vi "LuaVIEW Pushing and Pulling.vi"() -> (0 "pass?":bool)   [LabVIEW 2012]
uses:
  typedefs/t_LuaVIEW Reference.ctl
  subvis/private/LuaVIEW Pull (boolean).vi
  subvis/private/LuaVIEW Push (boolean).vi
  subvis/private/LuaVIEW Pull (number).vi
  subvis/private/LuaVIEW Push (number).vi
  subvis/private/LuaVIEW Pull (string).vi
  subvis/private/LuaVIEW Push (string).vi
  subvis/private/LuaVIEW Pull (path).vi
  subvis/private/LuaVIEW Push (path).vi
  subvis/private/LuaVIEW Pull (U32).vi
  subvis/private/LuaVIEW Push (object).vi
  subvis/private/LuaVIEW Pull (object).vi
  subvis/private/LuaVIEW Push (U32).vi
  subvis/private/LuaVIEW Push (refnum).vi
  subvis/private/LuaVIEW Pull (refnum).vi
  subvis/private/LuaVIEW Pull (I8).vi
  subvis/private/LuaVIEW Push (I8).vi
  subvis/private/LuaVIEW Pull (U8).vi
  subvis/private/LuaVIEW Push (U8).vi
  subvis/private/LuaVIEW Pull (I16).vi
  subvis/private/LuaVIEW Push (I16).vi
  subvis/private/LuaVIEW Pull (U16).vi
  subvis/private/LuaVIEW Push (U16).vi
  subvis/private/LuaVIEW Pull (I32).vi
  subvis/private/LuaVIEW Push (I32).vi
panel:
  in  "script file":path=path "scripts/push pull test.lua"
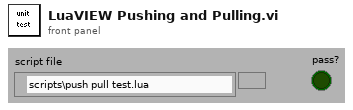
[diagram p1: front panel]
types:
  T1 = enum32{"execute", "initialize", "bool:b=pass_boolean(bool:b)", "pull_boolean(any:value)", "num:n=pass_number(num:n)", "pull_number(any:value)", "str:s=pass_string(str:s)", "pull_string(any:value)", "str:s=pass_path(str:s)", "pull_path(any:value)", "obj:o=push_object(U32:u,str:methodtable)", "U32:u=pull_object(any:value)", "bool:already_dead=kill_object(obj:o)", "any:attribute=get_object_attribute(str:key,obj:o)", "set_object_attribute(str:key,obj:o,any:value)", "any:attribute=unchecked_goa(any:key,...)", "unchecked_soa(any:key,...)", "ref:r=push_refnum(U32:u)", "U32:u=pull_refnum(any:value)", "I8:n=pass_I8(I8:n)", "pull_I8(any:value)", "U8:n=pass_U8(U8:n)", "pull_U8(any:value)", "I16:n=pass_I16(I16:n)", "pull_I16(any:value)", "U16:n=pass_U16(U16:n)", "pull_U16(any:value)", "I32:n=pass_I32(I32:n)", "pull_I32(any:value)", "U32:n=pass_U32(U32:n)", "pull_U32(any:value)", "str:buf=dump()", "str:new,I32:index=poll(I32:index)", "cleanup"}
  T2 = typedef "t_LuaVIEW Reference.ctl" = refnum<k1>
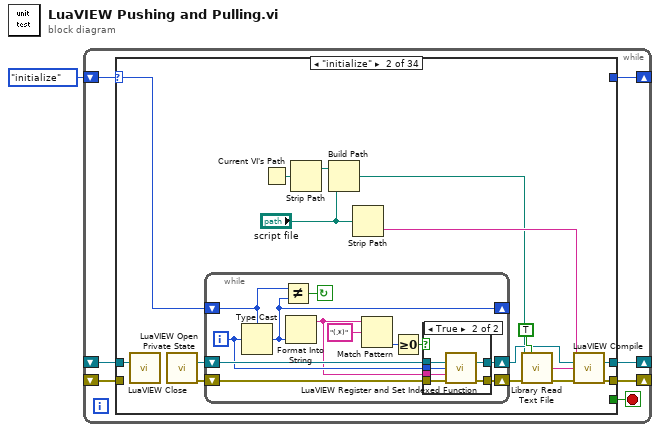
[diagram p0: block diagram]
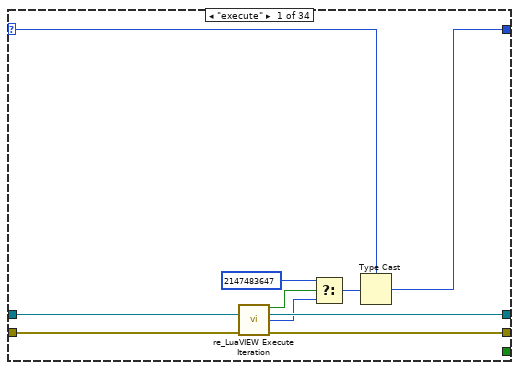
[diagram p2: hidden frame]
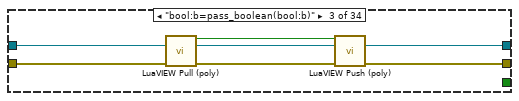
[diagram p4: hidden frame]
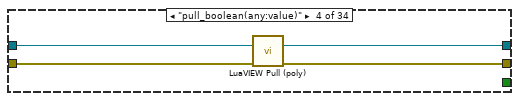
[diagram p5: hidden frame]
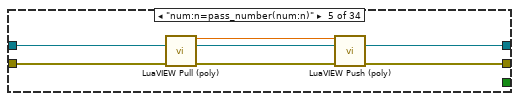
[diagram p6: hidden frame]
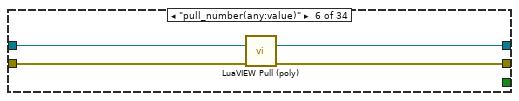
[diagram p7: hidden frame]
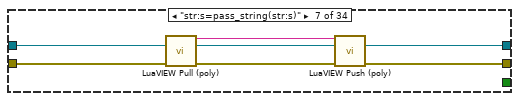
[diagram p8: hidden frame]
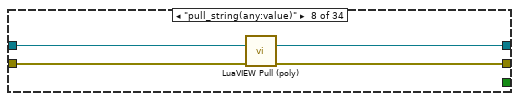
[diagram p9: hidden frame]
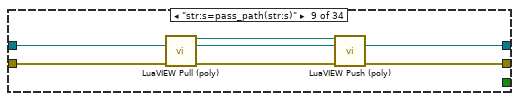
[diagram p10: hidden frame]
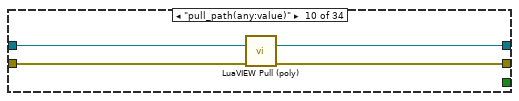
[diagram p11: hidden frame]
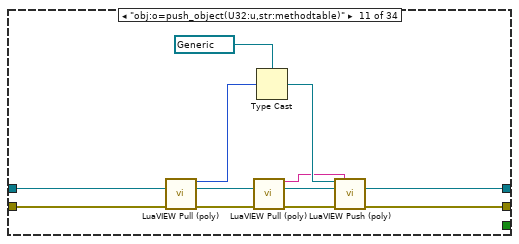
[diagram p12: hidden frame]
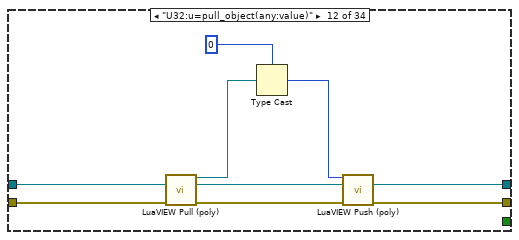
[diagram p13: hidden frame]
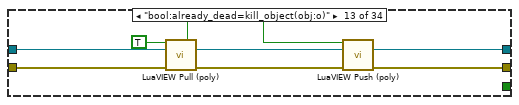
[diagram p14: hidden frame]
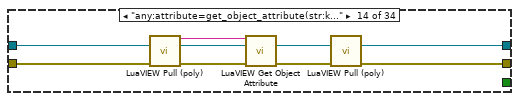
[diagram p15: hidden frame]
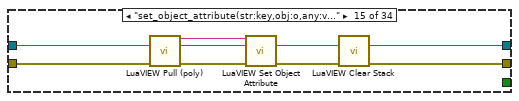
[diagram p16: hidden frame]
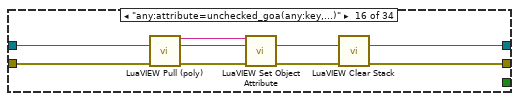
[diagram p17: hidden frame]
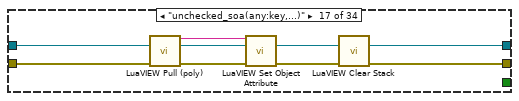
[diagram p18: hidden frame]
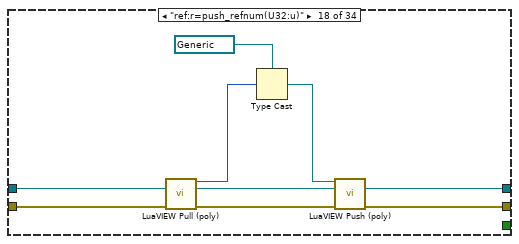
[diagram p19: hidden frame]
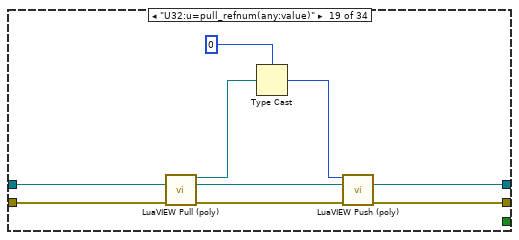
[diagram p20: hidden frame]
diagram:
  n1 = while {
    shift-right: [w6] -> _
    shift-left: T1."initialize" -> [w8]
    shift-right: [w4] -> _
    shift-left: _ -> [w5]
    shift-right: [w3] -> _
    shift-left: _ -> [w2]
    stop <- w7 stop-if-true
    n2 = case shown="\"initialize\"" w8 {
      selector: w8 -> [w11 w30 _ _ _ _ _ _ _ _ _ _ _ _ _ _ _ _ _ _ _ _ _ _ _ _ _ _ _ _ _ _ _ _]
      tunnel: [_ _ _ _ _ _ _ _ _ _ _ _ _ _ _ _ _ _ _ _ _ _ _ _ _ _ _ _ _ _ _ _ _ TRUE] -> w7
      tunnel: [w9 _ _ _ _ _ _ _ _ _ _ _ _ _ _ _ _ _ _ _ _ _ _ _ _ _ _ _ _ _ _ _ _ _] -> w6
      tunnel: w5 -> [w18 w34 w60 w64 w71 w75 w82 w86 w93 w97 w107 w118 w126 w135 w144 w153 w162 w169 w180 w187 w191 w198 w202 w209 w213 w220 w224 w231 w235 w242 w246 w254 w258 w276]
      tunnel: [w15 w31 w58 w62 w69 w73 w80 w85 w91 w96 w105 w115 w124 w128 w137 w146 w155 w166 w177 w185 w190 w196 w201 w207 w212 w218 w223 w229 w234 w240 w245 w248 w262 w275] -> w4
      tunnel: [w16 w29 w57 w63 w68 w74 w79 w84 w90 w95 w104 w114 w123 w129 w138 w147 w156 w165 w176 w184 w189 w195 w200 w206 w211 w217 w222 w228 w233 w239 w244 w251 w261 _] -> w3
      tunnel: w2 -> [w17 _ w61 w65 w72 w76 w83 w87 w94 w98 w108 w119 w127 w136 w145 w154 w163 w170 w181 w188 w192 w199 w203 w210 w214 w221 w225 w232 w236 w243 w247 w255 w260 w273]
      frame "execute" {
        n3 = call "re_LuaVIEW Execute Iteration.vi"("LuaVIEW reference in"=w18, "init or indexed function error"=w17) -> ("last?"=w13:bool, "LuaVIEW reference out"=w15:T2, "function index"=w14:i32, "final error"=w16:errorcluster)  [unwired: 10 in]
        n4 = Select(t=2147483647, s=w13, f=w14) -> (s? t:f=w10:i32)
        n5 = Type Cast(type=w11, x=w10) -> (*(type *) &x=w9:T1)
      }
      frame "initialize" {
        n6 = call "LuaVIEW Close.vi"("LuaVIEW reference"=w34) -> ()  [unwired: 14 in, 1 out]
        n7 = call "LuaVIEW Open Private State.vi"() -> ("LuaVIEW reference"=w32:T2, "error out"=w33:errorcluster)  [unwired: 14 in]
        n8 = while {
          shift-right: [w40] -> w25
          shift-left: w33 -> [w43]
          shift-right: [w41] -> w26
          shift-left: w32 -> [w42]
          shift-right: [w35] -> _
          shift-left: w30 -> [w36]
          i -> [w39]
          stop <- w46 continue-if-true
          n9 = Type Cast(type=w36, x=w39) -> (*(type *) &x=w35:T1)
          n10 = Not Equal?(x=w36, y=w35) -> (x != y?=w46:bool)
          n11 = Format Into String(w35) -> (resulting string=w37:string)  [unwired: 3 in, 1 out]
          n12 = Match Pattern(string=w37, regular expression="(.*)") -> (offset past match=w44:i32)  [unwired: 1 in, 3 out]
          n13 = Greater Or Equal To 0?(x=w44) -> (x >= 0?=w38:bool)
          n14 = case shown="True" w38 {
            tunnel: w42 -> [w48 w51]
            tunnel: w39 -> [_ w52]
            tunnel: w37 -> [_ w49]
            tunnel: [w47 w54] -> w40
            tunnel: [w48 w53] -> w41
            tunnel: w43 -> [w47 w50]
            frame False {
            }
            frame True {
              n15 = call "LuaVIEW Register and Set Indexed Function.vi"("LuaVIEW reference in"=w51, "index"=w52, "synopsis"=w49, "error in (no error)"=w50) -> ("LuaVIEW reference out"=w53:T2, "error out"=w54:errorcluster)  [unwired: 10 in]
            }
          }
        }
        n16 = Current VI's Path() -> (path=w23:path)
        n17 = Strip Path(path=w23) -> (stripped path=w22:path)  [unwired: 1 out]
        n18 = Build Path(base path=w22, name or relative path="script file") -> (appended path=w19:path)
        n19 = Strip Path(path="script file") -> (name=w20:string)  [unwired: 1 out]
        n20 = call "Library Read Text File.vi"("file path"=w19, "convert eol (F)"=TRUE, "error in (no error)"=w25) -> ("read text"=w24:string, "error out"=w27:errorcluster)  [unwired: 10 in, 1 out]
        n21 = call "LuaVIEW Compile.vi"("script name"=w20, "LuaVIEW reference in"=w26, "script"=w24, "error in (no error)"=w27) -> ("LuaVIEW reference out"=w31:T2, "error out"=w29:errorcluster)  [unwired: 10 in]
      }
      frame "bool:b=pass_boolean(bool:b)" {
        n22 = call-poly "LuaVIEW Pull (poly).vi"("LuaVIEW reference in"=w60, "error in (no error)"=w61) -> ("boolean"=w55:bool, "LuaVIEW reference out"=w56:T2, "error out"=w59:errorcluster)  [unwired: 11 in]
        n23 = call-poly "LuaVIEW Push (poly).vi"("boolean"=w55, "LuaVIEW reference in"=w56, "error in (no error)"=w59) -> ("LuaVIEW reference out"=w58:T2, "error out"=w57:errorcluster)  [unwired: 11 in]
      }
      frame "pull_boolean(any:value)" {
        n24 = call-poly "LuaVIEW Pull (poly).vi"("LuaVIEW reference in"=w64, "error in (no error)"=w65) -> ("LuaVIEW reference out"=w62:T2, "error out"=w63:errorcluster)  [unwired: 11 in, 1 out]
      }
      frame "num:n=pass_number(num:n)" {
        n25 = call-poly "LuaVIEW Pull (poly).vi"("LuaVIEW reference in"=w71, "error in (no error)"=w72) -> ("number"=w66:dbl, "LuaVIEW reference out"=w67:T2, "error out"=w70:errorcluster)  [unwired: 11 in]
        n26 = call-poly "LuaVIEW Push (poly).vi"("number"=w66, "LuaVIEW reference in"=w67, "error in (no error)"=w70) -> ("LuaVIEW reference out"=w69:T2, "error out"=w68:errorcluster)  [unwired: 11 in]
      }
      frame "pull_number(any:value)" {
        n27 = call-poly "LuaVIEW Pull (poly).vi"("LuaVIEW reference in"=w75, "error in (no error)"=w76) -> ("LuaVIEW reference out"=w73:T2, "error out"=w74:errorcluster)  [unwired: 11 in, 1 out]
      }
      frame "str:s=pass_string(str:s)" {
        n28 = call-poly "LuaVIEW Pull (poly).vi"("LuaVIEW reference in"=w82, "error in (no error)"=w83) -> ("string"=w77:string, "LuaVIEW reference out"=w78:T2, "error out"=w81:errorcluster)  [unwired: 11 in]
        n29 = call-poly "LuaVIEW Push (poly).vi"("string"=w77, "LuaVIEW reference in"=w78, "error in (no error)"=w81) -> ("LuaVIEW reference out"=w80:T2, "error out"=w79:errorcluster)  [unwired: 11 in]
      }
      frame "pull_string(any:value)" {
        n30 = call-poly "LuaVIEW Pull (poly).vi"("LuaVIEW reference in"=w86, "error in (no error)"=w87) -> ("LuaVIEW reference out"=w85:T2, "error out"=w84:errorcluster)  [unwired: 11 in, 1 out]
      }
      frame "str:s=pass_path(str:s)" {
        n31 = call-poly "LuaVIEW Pull (poly).vi"("LuaVIEW reference in"=w93, "error in (no error)"=w94) -> ("path"=w88:path, "LuaVIEW reference out"=w89:T2, "error out"=w92:errorcluster)  [unwired: 11 in]
        n32 = call-poly "LuaVIEW Push (poly).vi"("path"=w88, "LuaVIEW reference in"=w89, "error in (no error)"=w92) -> ("LuaVIEW reference out"=w91:T2, "error out"=w90:errorcluster)  [unwired: 11 in]
      }
      frame "pull_path(any:value)" {
        n33 = call-poly "LuaVIEW Pull (poly).vi"("LuaVIEW reference in"=w97, "error in (no error)"=w98) -> ("LuaVIEW reference out"=w96:T2, "error out"=w95:errorcluster)  [unwired: 11 in, 1 out]
      }
      frame "obj:o=push_object(U32:u,str:methodtable)" {
        n34 = call-poly "LuaVIEW Pull (poly).vi"("LuaVIEW reference in"=w107, "error in (no error)"=w108) -> ("U32"=w106:u32, "LuaVIEW reference out"=w102:T2, "error out"=w103:errorcluster)  [unwired: 11 in]
        n35 = call-poly "LuaVIEW Pull (poly).vi"("LuaVIEW reference in"=w102, "error in (no error)"=w103) -> ("string"=w99:string, "LuaVIEW reference out"=w100:T2, "error out"=w101:errorcluster)  [unwired: 11 in]
        n36 = Type Cast(type=refnum<vi> refnum ("refnum"), x=w106) -> (*(type *) &x=w109:refnum<vi>)
        n37 = call-poly "LuaVIEW Push (poly).vi"("object refnum"=w109, "method table (use caller's function table)"=w99, "LuaVIEW reference in"=w100, "error in (no error)"=w101) -> ("LuaVIEW reference out"=w105:T2, "error out"=w104:errorcluster)  [unwired: 10 in]
      }
      frame "U32:u=pull_object(any:value)" {
        n38 = call-poly "LuaVIEW Pull (poly).vi"("LuaVIEW reference in"=w118, "error in (no error)"=w119) -> ("object refnum"=w116:refnum<vi>, "LuaVIEW reference out"=w113:T2, "error out"=w117:errorcluster)  [unwired: 10 in, 1 out]
        n39 = Type Cast(type=u32 0 ("U32"), x=w116) -> (*(type *) &x=w111:u32)
        n40 = call-poly "LuaVIEW Push (poly).vi"("U32"=w111, "LuaVIEW reference in"=w113, "error in (no error)"=w117) -> ("LuaVIEW reference out"=w115:T2, "error out"=w114:errorcluster)  [unwired: 11 in]
      }
      frame "bool:already_dead=kill_object(obj:o)" {
        n41 = call-poly "LuaVIEW Pull (poly).vi"("kill (false)"=TRUE, "LuaVIEW reference in"=w126, "error in (no error)"=w127) -> ("already dead?"=w120:bool, "LuaVIEW reference out"=w122:T2, "error out"=w125:errorcluster)  [unwired: 9 in, 1 out]
        n42 = call-poly "LuaVIEW Push (poly).vi"("boolean"=w120, "LuaVIEW reference in"=w122, "error in (no error)"=w125) -> ("LuaVIEW reference out"=w124:T2, "error out"=w123:errorcluster)  [unwired: 11 in]
      }
      frame "any:attribute=get_object_attribute(str:key,obj:o)" {
        n43 = call-poly "LuaVIEW Pull (poly).vi"("LuaVIEW reference in"=w135, "error in (no error)"=w136) -> ("string"=w132:string, "LuaVIEW reference out"=w133:T2, "error out"=w134:errorcluster)  [unwired: 11 in]
        n44 = call "LuaVIEW Get Object Attribute.vi"("key"=w132, "LuaVIEW reference in"=w133, "error in (no error)"=w134) -> ("LuaVIEW reference out"=w130:T2, "error out"=w131:errorcluster)  [unwired: 11 in]
        n45 = call-poly "LuaVIEW Pull (poly).vi"("LuaVIEW reference in"=w130, "error in (no error)"=w131) -> ("LuaVIEW reference out"=w128:T2, "error out"=w129:errorcluster)  [unwired: 10 in, 2 out]
      }
      frame "set_object_attribute(str:key,obj:o,any:value)" {
        n46 = call-poly "LuaVIEW Pull (poly).vi"("LuaVIEW reference in"=w144, "error in (no error)"=w145) -> ("string"=w141:string, "LuaVIEW reference out"=w142:T2, "error out"=w143:errorcluster)  [unwired: 11 in]
        n47 = call "LuaVIEW Set Object Attribute.vi"("key"=w141, "LuaVIEW reference in"=w142, "error in (no error)"=w143) -> ("LuaVIEW reference out"=w139:T2, "error out"=w140:errorcluster)  [unwired: 11 in]
        n48 = call "LuaVIEW Clear Stack.vi"("LuaVIEW reference in"=w139, "error in (no error)"=w140) -> ("LuaVIEW reference out"=w137:T2, "error out"=w138:errorcluster)  [unwired: 12 in]
      }
      frame "any:attribute=unchecked_goa(any:key,...)" {
        n49 = call-poly "LuaVIEW Pull (poly).vi"("LuaVIEW reference in"=w153, "error in (no error)"=w154) -> ("string"=w150:string, "LuaVIEW reference out"=w151:T2, "error out"=w152:errorcluster)  [unwired: 11 in]
        n50 = call "LuaVIEW Set Object Attribute.vi"("key"=w150, "LuaVIEW reference in"=w151, "error in (no error)"=w152) -> ("LuaVIEW reference out"=w148:T2, "error out"=w149:errorcluster)  [unwired: 11 in]
        n51 = call "LuaVIEW Clear Stack.vi"("LuaVIEW reference in"=w148, "error in (no error)"=w149) -> ("LuaVIEW reference out"=w146:T2, "error out"=w147:errorcluster)  [unwired: 12 in]
      }
      frame "unchecked_soa(any:key,...)" {
        n52 = call-poly "LuaVIEW Pull (poly).vi"("LuaVIEW reference in"=w162, "error in (no error)"=w163) -> ("string"=w159:string, "LuaVIEW reference out"=w160:T2, "error out"=w161:errorcluster)  [unwired: 11 in]
        n53 = call "LuaVIEW Set Object Attribute.vi"("key"=w159, "LuaVIEW reference in"=w160, "error in (no error)"=w161) -> ("LuaVIEW reference out"=w157:T2, "error out"=w158:errorcluster)  [unwired: 11 in]
        n54 = call "LuaVIEW Clear Stack.vi"("LuaVIEW reference in"=w157, "error in (no error)"=w158) -> ("LuaVIEW reference out"=w155:T2, "error out"=w156:errorcluster)  [unwired: 12 in]
      }
      frame "ref:r=push_refnum(U32:u)" {
        n55 = call-poly "LuaVIEW Pull (poly).vi"("LuaVIEW reference in"=w169, "error in (no error)"=w170) -> ("U32"=w167:u32, "LuaVIEW reference out"=w164:T2, "error out"=w168:errorcluster)  [unwired: 11 in]
        n56 = Type Cast(type=refnum<vi> refnum ("refnum"), x=w167) -> (*(type *) &x=w171:refnum<vi>)
        n57 = call-poly "LuaVIEW Push (poly).vi"("refnum"=w171, "LuaVIEW reference in"=w164, "error in (no error)"=w168) -> ("LuaVIEW reference out"=w166:T2, "error out"=w165:errorcluster)  [unwired: 11 in]
      }
      frame "U32:u=pull_refnum(any:value)" {
        n58 = call-poly "LuaVIEW Pull (poly).vi"("LuaVIEW reference in"=w180, "error in (no error)"=w181) -> ("refnum"=w178:refnum<vi>, "LuaVIEW reference out"=w175:T2, "error out"=w179:errorcluster)  [unwired: 11 in]
        n59 = Type Cast(type=u32 0 ("U32"), x=w178) -> (*(type *) &x=w173:u32)
        n60 = call-poly "LuaVIEW Push (poly).vi"("U32"=w173, "LuaVIEW reference in"=w175, "error in (no error)"=w179) -> ("LuaVIEW reference out"=w177:T2, "error out"=w176:errorcluster)  [unwired: 11 in]
      }
      frame "I8:n=pass_I8(I8:n)" {
        n61 = call-poly "LuaVIEW Pull (poly).vi"("LuaVIEW reference in"=w187, "error in (no error)"=w188) -> ("I8"=w182:i8, "LuaVIEW reference out"=w183:T2, "error out"=w186:errorcluster)  [unwired: 11 in]
        n62 = call-poly "LuaVIEW Push (poly).vi"("I8"=w182, "LuaVIEW reference in"=w183, "error in (no error)"=w186) -> ("LuaVIEW reference out"=w185:T2, "error out"=w184:errorcluster)  [unwired: 11 in]
      }
      frame "pull_I8(any:value)" {
        n63 = call-poly "LuaVIEW Pull (poly).vi"("LuaVIEW reference in"=w191, "error in (no error)"=w192) -> ("LuaVIEW reference out"=w190:T2, "error out"=w189:errorcluster)  [unwired: 11 in, 1 out]
      }
      frame "U8:n=pass_U8(U8:n)" {
        n64 = call-poly "LuaVIEW Pull (poly).vi"("LuaVIEW reference in"=w198, "error in (no error)"=w199) -> ("U8"=w193:u8, "LuaVIEW reference out"=w194:T2, "error out"=w197:errorcluster)  [unwired: 11 in]
        n65 = call-poly "LuaVIEW Push (poly).vi"("U8"=w193, "LuaVIEW reference in"=w194, "error in (no error)"=w197) -> ("LuaVIEW reference out"=w196:T2, "error out"=w195:errorcluster)  [unwired: 11 in]
      }
      frame "pull_U8(any:value)" {
        n66 = call-poly "LuaVIEW Pull (poly).vi"("LuaVIEW reference in"=w202, "error in (no error)"=w203) -> ("LuaVIEW reference out"=w201:T2, "error out"=w200:errorcluster)  [unwired: 11 in, 1 out]
      }
      frame "I16:n=pass_I16(I16:n)" {
        n67 = call-poly "LuaVIEW Pull (poly).vi"("LuaVIEW reference in"=w209, "error in (no error)"=w210) -> ("I16"=w204:i16, "LuaVIEW reference out"=w205:T2, "error out"=w208:errorcluster)  [unwired: 11 in]
        n68 = call-poly "LuaVIEW Push (poly).vi"("I16"=w204, "LuaVIEW reference in"=w205, "error in (no error)"=w208) -> ("LuaVIEW reference out"=w207:T2, "error out"=w206:errorcluster)  [unwired: 11 in]
      }
      frame "pull_I16(any:value)" {
        n69 = call-poly "LuaVIEW Pull (poly).vi"("LuaVIEW reference in"=w213, "error in (no error)"=w214) -> ("LuaVIEW reference out"=w212:T2, "error out"=w211:errorcluster)  [unwired: 11 in, 1 out]
      }
      frame "U16:n=pass_U16(U16:n)" {
        n70 = call-poly "LuaVIEW Pull (poly).vi"("LuaVIEW reference in"=w220, "error in (no error)"=w221) -> ("U16"=w215:u16, "LuaVIEW reference out"=w216:T2, "error out"=w219:errorcluster)  [unwired: 11 in]
        n71 = call-poly "LuaVIEW Push (poly).vi"("U16"=w215, "LuaVIEW reference in"=w216, "error in (no error)"=w219) -> ("LuaVIEW reference out"=w218:T2, "error out"=w217:errorcluster)  [unwired: 11 in]
      }
      frame "pull_U16(any:value)" {
        n72 = call-poly "LuaVIEW Pull (poly).vi"("LuaVIEW reference in"=w224, "error in (no error)"=w225) -> ("LuaVIEW reference out"=w223:T2, "error out"=w222:errorcluster)  [unwired: 11 in, 1 out]
      }
      frame "I32:n=pass_I32(I32:n)" {
        n73 = call-poly "LuaVIEW Pull (poly).vi"("LuaVIEW reference in"=w231, "error in (no error)"=w232) -> ("I32"=w226:i32, "LuaVIEW reference out"=w227:T2, "error out"=w230:errorcluster)  [unwired: 11 in]
        n74 = call-poly "LuaVIEW Push (poly).vi"("I32"=w226, "LuaVIEW reference in"=w227, "error in (no error)"=w230) -> ("LuaVIEW reference out"=w229:T2, "error out"=w228:errorcluster)  [unwired: 11 in]
      }
      frame "pull_I32(any:value)" {
        n75 = call-poly "LuaVIEW Pull (poly).vi"("LuaVIEW reference in"=w235, "error in (no error)"=w236) -> ("LuaVIEW reference out"=w234:T2, "error out"=w233:errorcluster)  [unwired: 11 in, 1 out]
      }
      frame "U32:n=pass_U32(U32:n)" {
        n76 = call-poly "LuaVIEW Pull (poly).vi"("LuaVIEW reference in"=w242, "error in (no error)"=w243) -> ("U32"=w237:u32, "LuaVIEW reference out"=w238:T2, "error out"=w241:errorcluster)  [unwired: 11 in]
        n77 = call-poly "LuaVIEW Push (poly).vi"("U32"=w237, "LuaVIEW reference in"=w238, "error in (no error)"=w241) -> ("LuaVIEW reference out"=w240:T2, "error out"=w239:errorcluster)  [unwired: 11 in]
      }
      frame "pull_U32(any:value)" {
        n78 = call-poly "LuaVIEW Pull (poly).vi"("LuaVIEW reference in"=w246, "error in (no error)"=w247) -> ("LuaVIEW reference out"=w245:T2, "error out"=w244:errorcluster)  [unwired: 11 in, 1 out]
      }
      frame "str:buf=dump()" {
        n79 = call "LuaVIEW Poll Print Buffer.vi"("LuaVIEW reference in"=w254, "read all?"=TRUE, "error in (no error)"=w255) -> ("text"=w250:string, "LuaVIEW reference out"=w249:T2, "error out"=w252:errorcluster)  [unwired: 8 in, 2 out]
        n80 = call-poly "LuaVIEW Push (poly).vi"("string"=w250, "LuaVIEW reference in"=w249, "error in (no error)"=w252) -> ("LuaVIEW reference out"=w248:T2, "error out"=w251:errorcluster)  [unwired: 11 in]
      }
      frame "str:new,I32:index=poll(I32:index)" {
        n81 = call-poly "LuaVIEW Pull (poly).vi"("LuaVIEW reference in"=w258, "error in (no error)"=w260) -> ("I32"=w256:i32, "LuaVIEW reference out"=w257:T2, "error out"=w259:errorcluster)  [unwired: 11 in]
        n82 = call "LuaVIEW Poll Print Buffer.vi"("LuaVIEW reference in"=w257, "read all?"=FALSE, "read index in"=w256, "error in (no error)"=w259) -> ("text"=w267:string, "LuaVIEW reference out"=w266:T2, "read index out"=w263:i32, "error out"=w268:errorcluster)  [unwired: 7 in, 1 out]
        n83 = call-poly "LuaVIEW Push (poly).vi"("string"=w267, "LuaVIEW reference in"=w266, "error in (no error)"=w268) -> ("LuaVIEW reference out"=w264:T2, "error out"=w265:errorcluster)  [unwired: 11 in]
        n84 = call-poly "LuaVIEW Push (poly).vi"("I32"=w263, "LuaVIEW reference in"=w264, "error in (no error)"=w265) -> ("LuaVIEW reference out"=w262:T2, "error out"=w261:errorcluster)  [unwired: 11 in]
      }
      frame "cleanup" {
        w275 = T2 refnum items=["LuaVIEW"] ("LuaVIEW reference")
        n85 = call "LuaVIEW Close.vi"("LuaVIEW reference"=w276, "error in (no error)"=w273) -> ("dup error"=w272:errorcluster)  [unwired: 13 in]
        n86 = call "Library Log Error to Window.vi"("error in (no error)"=w272) -> ("error?"=w271:bool)  [unwired: 13 in, 1 out]
        n87 = Not(x=w271) -> (.not. x?=→"pass?":bool)
      }
    }
  }
